vi "QDInstrument_OptiCool_Remote Control.vi"() -> ()   [LabVIEW 2021]
uses:
  <vilib>/Analysis/baseanly.llb/Mean (DBL).vi
  <vilib>/Analysis/NI_AALBase.lvlib
panel:
  in  "Field Approach":i32(ring) items=["Linear", "NoOvershoot", "Oscillate"]
  in  "Field Rate":dbl=50.0 format="%#_13g"
  in  "Set Field":dbl format="%#_13g"
  in  "Mode":i32(ring) items=["Persistent", "Driven"]
  in  "Temperature Approach":i32(ring) items=["FastSettle", "NoOvershoot"]
  in  "Temperautre Rate":dbl=20.0
  in  "Set  Temperature":dbl=300.0
  in  "WaitForField":bool=TRUE
  in  "WaitFor\nTemperature":bool=TRUE
  out "Temperature\nStatus":i32(ring) items=["TemperatureUnknown"=0, "Stable"=1, "Tracking"=2, "Near"=5, "Chasing"=6, "Filling"=7, "Standby"=10, "Disabled"=13, "ImpedanceNotFunction"=14, "TempFailure"=15]
  out "Field\nStatus":i32(ring) items=["MagnetUnknown"=0, "StablePersistent"=1, "WarmingSwitch"=2, "CoolingSwitch"=3, "StableDriven"=4, "Iterating"=5, "Charging"=6, "Discharging"=7, "CurrentError"=8, "MagnetFailure"=15]
  out "Field":dbl
  in  "Delay":dbl=5.0
  out "Temperature":dbl
  in  "Remote":bool=TRUE
  in  "IP Address":string="169.254.170.239"
  out "Measuring":bool
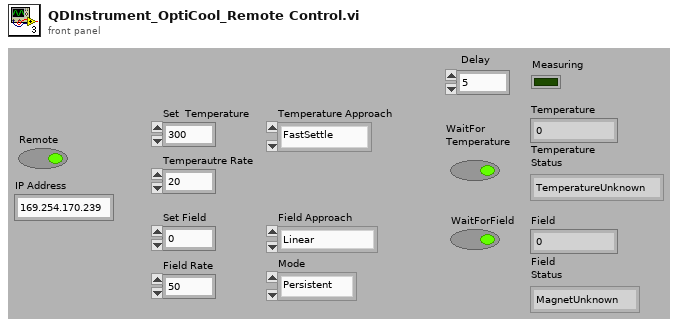
[diagram p1: front panel]
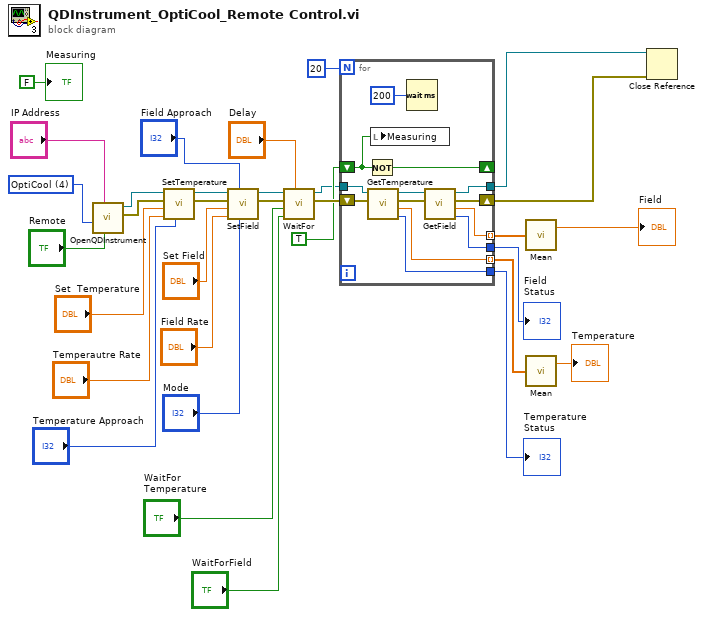
[diagram p0: block diagram]
diagram:
  w22 = 4 items=["PPMS", "VersaLab", "DynaCool", "SVSM", "OptiCool"] ("InstrumentType")
  n1 = call "OpenQDInstrument.vi"("Remote"="Remote", "IP Address"="IP Address", "InstrumentType"=w22) -> ("error out"=w9:errorcluster, "Instrument Ref"=w10:refnum<k24>)  [unwired: 5 in]
  n2 = call "SetTemperature.vi"("Approach"="Temperature Approach", "Rate"="Temperautre Rate", "Temperature"="Set  Temperature", "error in (no error)"=w9, "Instrument Ref In"=w10) -> ("error out"=w28:errorcluster, "Instrument Ref Out"=w27:refnum<k24>)  [unwired: 2 in, 1 out]
  n3 = call "SetField.vi"("Mode"="Mode", "Approach"="Field Approach", "Rate"="Field Rate", "Field"="Set Field", "error in (no error)"=w28, "Instrument Ref In"=w27) -> ("error out"=w5:errorcluster, "Instrument Ref Out"=w6:refnum<k24>)  [unwired: 1 in, 1 out]
  n4 = call "WaitFor.vi"("Delay"="Delay", "Wait For Field"="WaitForField", "Wait For Temperature"="WaitFor\nTemperature", "error in (no error)"=w5, "Instrument Ref In"=w6) -> ("error out"=w21:errorcluster, "Instrument Ref Out"=w17:refnum<k24>)  [unwired: 5 in]
  n5 = for {
    N: 20 -> [_]
    shift-right: [w45] -> _
    shift-left: TRUE -> [w43]
    shift-right: [w40] -> w7
    shift-left: w21 -> [w42]
    tunnel: w17 -> [w39]
    tunnel: [w37] -> w8
    tunnel: [w34] -> w16
    tunnel: [w33] -> w15
    tunnel: [w35] -> w13 mode=indexing
    tunnel: [w36] -> w14 mode=indexing
    n6 = Not(x=w43) -> (.not. x?=w45:bool)
    n7 = call "GetTemperature.vi"("error in (no error)"=w42, "Instrument Ref In"=w39) -> ("Temperature\nStatus"=w33:i32, "Temperature"=w36:dbl, "error out"=w41:errorcluster, "Instrument Ref Out"=w38:refnum<k24>)  [unwired: 3 in, 1 out]
    n8 = local write "Measuring"(w43) -> ()
    n9 = Wait (ms)(milliseconds to wait=u32 200) -> ()  [unwired: 1 out]
    n10 = call "GetField.vi"("error in (no error)"=w41, "Instrument Ref In"=w38) -> ("Field\nStatus"=w34:i32, "Field"=w35:dbl, "error out"=w40:errorcluster, "Instrument Ref Out"=w37:refnum<k24>)  [unwired: 3 in, 1 out]
  }
  "Field\nStatus" <- w16
  "Temperature\nStatus" <- w15
  n11 = call-poly <vilib>:"Mean.vi"("X"=w13) -> ("mean"=→"Field":dbl)  [unwired: 1 out]
  n12 = call-poly <vilib>:"Mean.vi"("X"=w14) -> ("mean"=→"Temperature":dbl)  [unwired: 1 out]
  n13 = Close Reference(reference=w8, error in (no error)=w7) -> ()  [unwired: 1 out]
  "Measuring" <- FALSE
